vi "Grab and Attributes Setup with Save.vi"(8 "error in":errorcluster, 10 "Set Points":dbl[](array[numeric])=[1.0, 5.0, -0.1, 50.0]) -> (0 "error out":errorcluster)   [LabVIEW 2015]
doc: "The Grab and Attributes Setup example VI allows the user to view the current attributes and settings, update attribute settings, acquire images continuously, and display the images in an image control."
uses:
  <vilib>/vision/driver/IMAQdx.llb/IMAQdx Acquisition Mode.ctl
  <vilib>/vision/driver/IMAQdx.llb/IMAQdx Buffer Number Mode.ctl
  <vilib>/userDefined/High Color/IMAQdx.ctl
panel:
  in  "Cancel":bool
  in  "OK":bool
  in  "Tab Control 2":enum32{"Configure", "Help"}(tab)
  in  "Record images":bool
  in  "Image folder":path
  in  "Image Save Rate (s)":dbl=10.0 format="%#_5f"
  out "Interface elevation":dbl
  out "Camera Name":T1
  in  "Attribute Table":string(tree)
  in  "Tab Control":T2(tab)
  in  "U32 Value Control":u32(slide) min=480 max=921600 step=1 scale=829440.0..921600.0
  in  "DBL Value Control":dbl(slide) min=0.0 max=3.999 step=1.0 scale=0.0..3.999
  in  "String Value Control":string
  in  "Enum Value Control":u32(ring) items=["160x90 I420 15.00fps", "160x90 RGB24 15.00fps", "160x100 I420 15.00fps", "160x100 RGB24 15.00fps", "160x120 I420 15.00fps", "160x120 RGB24 15.00fps", "176x144 I420 15.00fps", "176x144 RGB24 15.00fps", "320x180 I420 15.00fps", "320x180 RGB24 15.00fps", "320x200 I420 15.00fps", "320x200 RGB24 15.00fps", "320x240 I420 15.00fps", "320x240 RGB24 15.00fps", "352x288 I420 15.00fps", "352x288 RGB24 15.00fps", "640x360 I420 15.00fps", "640x360 RGB24 15.00fps", "640x400 I420 15.00fps", "640x400 RGB24 15.00fps", "640x480 I420 30.00fps", "640x480 RGB24 30.00fps", "768x480 I420 15.00fps", "768x480 RGB24 15.00fps", "800x450 I420 15.00fps", "800x450 RGB24 15.00fps", "800x500 I420 15.00fps", "800x500 RGB24 15.00fps", "800x600 I420 15.00fps", "800x600 RGB24 15.00fps", "864x480 I420 15.00fps", "864x480 RGB24 15.00fps", "960x720 I420 15.00fps", "960x720 RGB24 15.00fps", "1280x720 I420 5.00fps", "1280x720 RGB24 5.00fps", "1280x800 I420 5.00fps", "1280x800 RGB24 5.00fps", "1280x1024 I420 5.00fps", "1280x1024 RGB24 5.00fps"]
  in  "Boolean Value Control":bool=TRUE
  in  "Command Value Control":bool
  out "Units":string
  out "Tooltip":string
  out "Image":T3(plugin-control)
  out "Buffer Number":u32
  out "Frame Rate":dbl(knob) scale=0.0..100.0 scale format="%.1f"
  in  "Grab":bool
  out "Tab Control Ref":T4
  # "Use the rectangle tool to define the region of interest where the floc water interface will appear.\nThe region of interest is saved in a configuration file.\n\nChoose a folder to save images during the experiment."
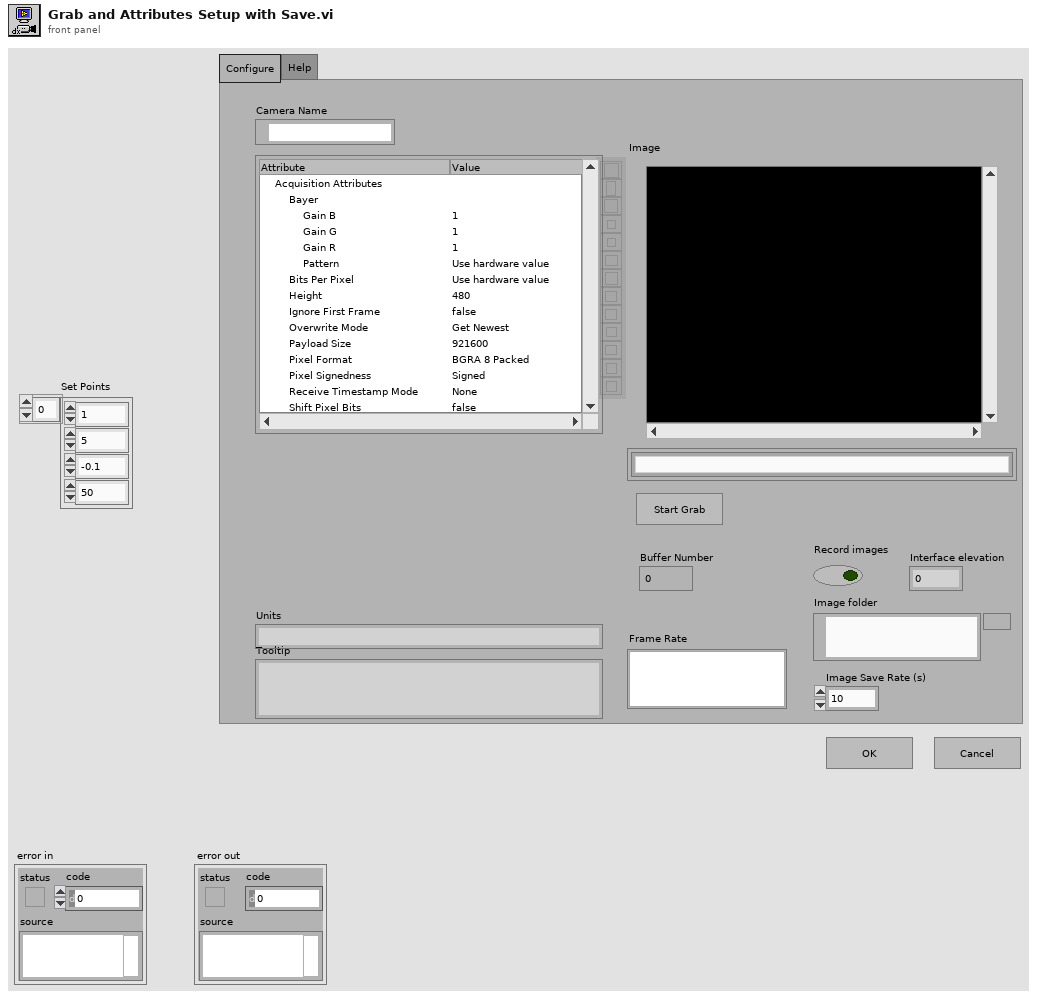
[diagram p1: front panel]
types:
  T1 = typedef "IMAQdx.ctl" = refnum<k21>
  T2 = enum32{"U32", "DBL", "String", "Enum", "Bool", "Command"}
  T3 = typedef "IMAQ Image.ctl" = refnum<image>
  T4 = cluster{"Tab Control":refnum<vi>, "U32 Value Control":refnum<vi>, "DBL Value Control":refnum<vi>, "String Value Control":refnum<vi>, "Enum Value Control":refnum<vi>, "Boolean Value Control":refnum<vi>, "Command Value Control":refnum<vi>}
  T5 = typedef "NI_Vision_Acquisition_Software.lvlib/IMAQdx Acquisition Mode.ctl" = enum32{"One Shot", "Continuous"}
  T6 = cluster{"Global Rectangle":i32[], "Contours":cluster{"Contour Type":u32, "ROI Type":u32, "Points":i32[]}[]}
  T7 = cluster{"Type":u32, "Version":u32, "Flags":u32, "SerialNumberHigh":u32, "SerialNumberLow":u32, "BusType":u32, "InterfaceName":string, "VendorName":string, "ModelName":string, "CameraFileName":string, "CameraAttributeURL":string}[]
  T8 = cluster{"Set Points[0]":dbl, "Set Points[1]":dbl, "Set Points[2]":dbl, "Set Points[3]":dbl}
  T9 = cluster{"Type":u32, "Version":u32, "Flags":u32, "SerialNumberHigh":u32, "SerialNumberLow":u32, "BusType":u32, "InterfaceName":string, "VendorName":string, "ModelName":string, "CameraFileName":string, "CameraAttributeURL":string}
  T10 = enum8{"Enabled", "Disabled", "Disabled and Grayed Out"}
  T11 = typedef "NI_Vision_Acquisition_Software.lvlib/IMAQdx Buffer Number Mode.ctl" = enum32{"Next", "Last", "Buffer Number"}
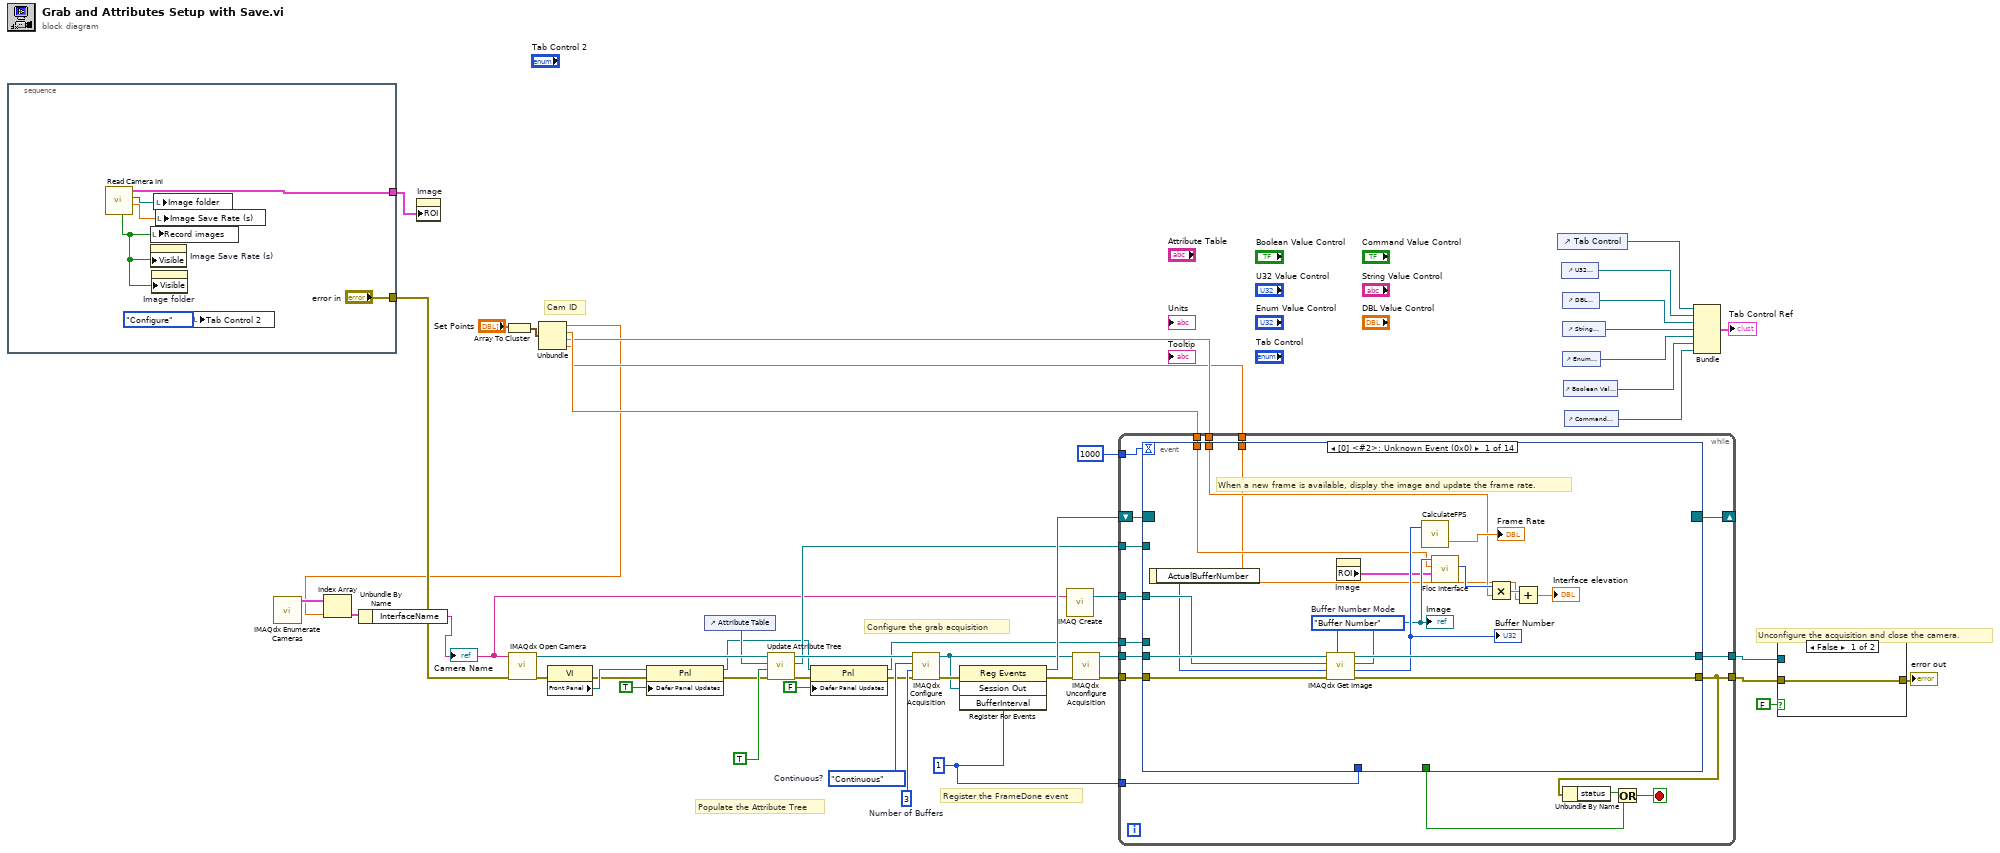
[diagram p0: block diagram]
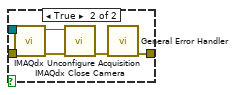
[diagram p2: hidden frame]
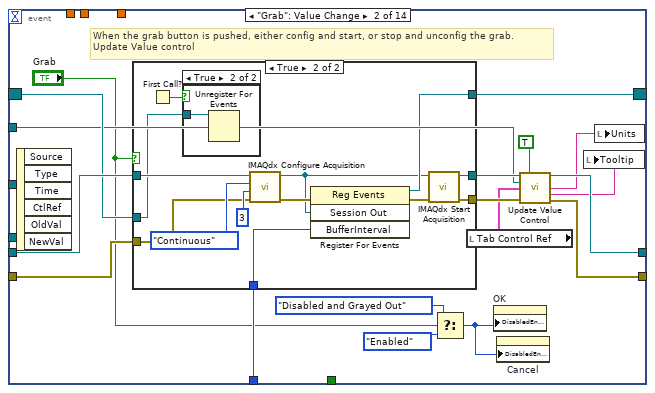
[diagram p3: hidden frame]
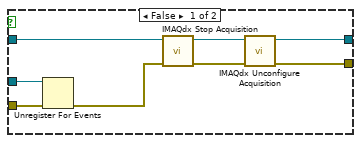
[diagram p4: hidden frame]
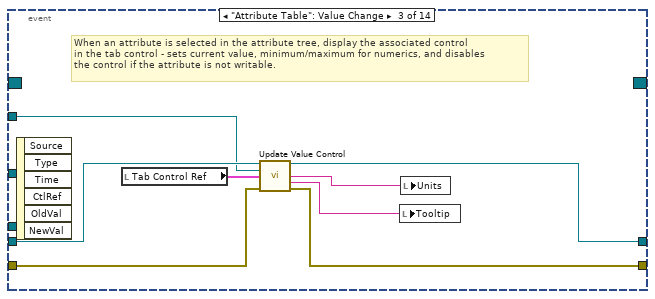
[diagram p6: hidden frame]
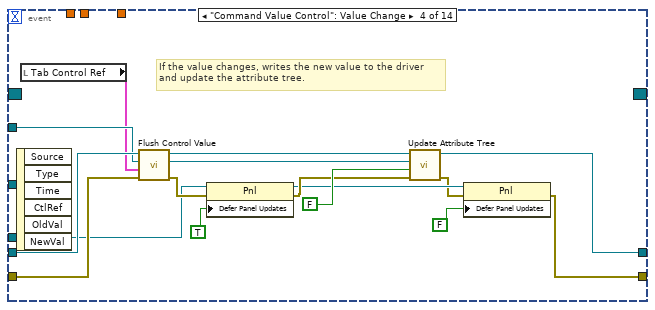
[diagram p7: hidden frame]
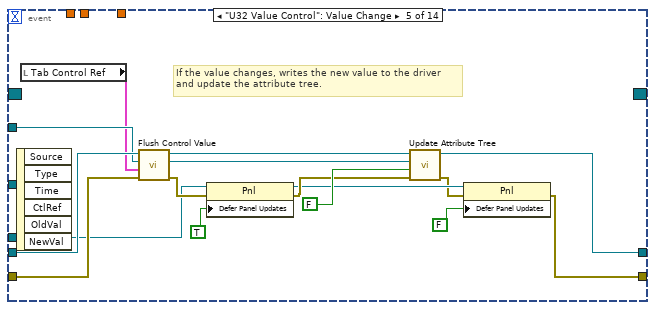
[diagram p8: hidden frame]
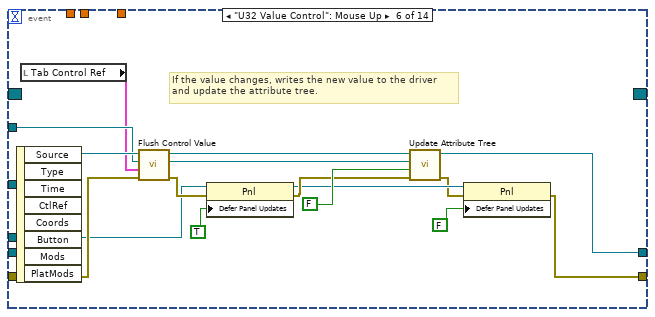
[diagram p9: hidden frame]
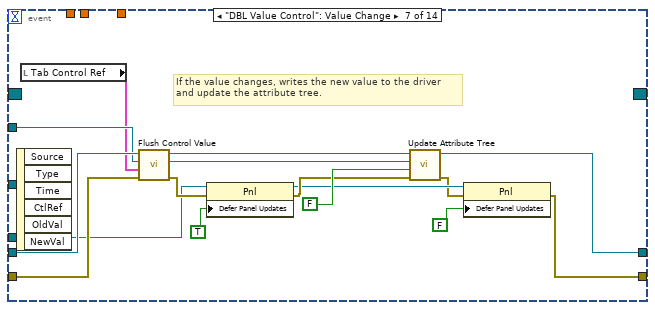
[diagram p10: hidden frame]
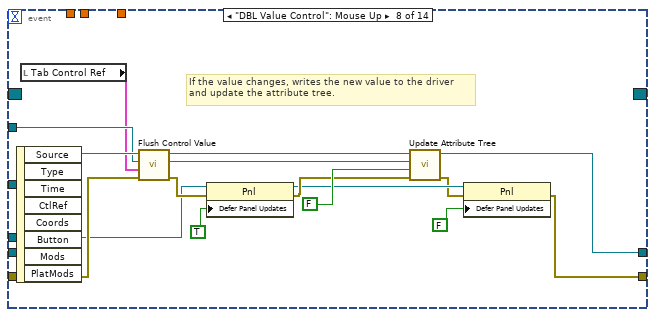
[diagram p11: hidden frame]
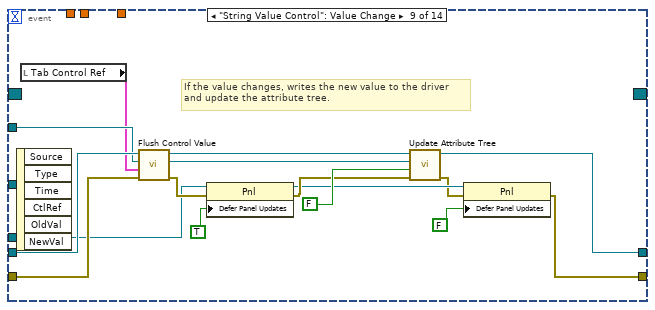
[diagram p12: hidden frame]
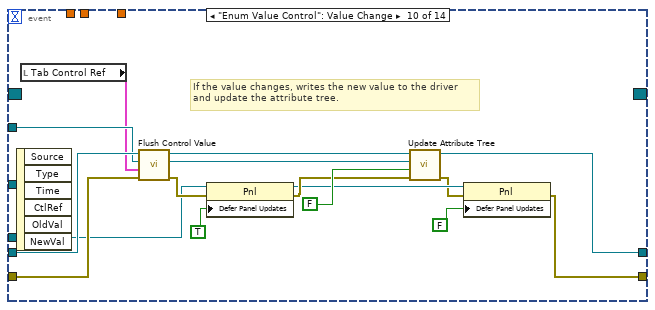
[diagram p13: hidden frame]
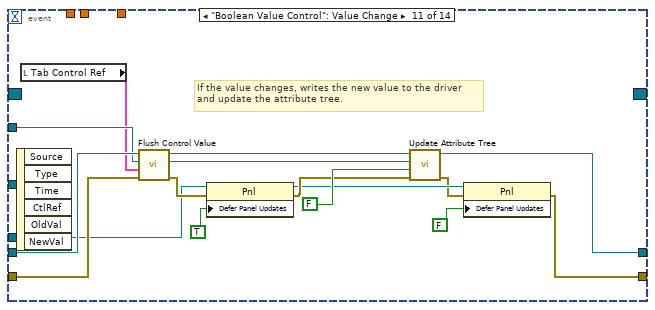
[diagram p14: hidden frame]
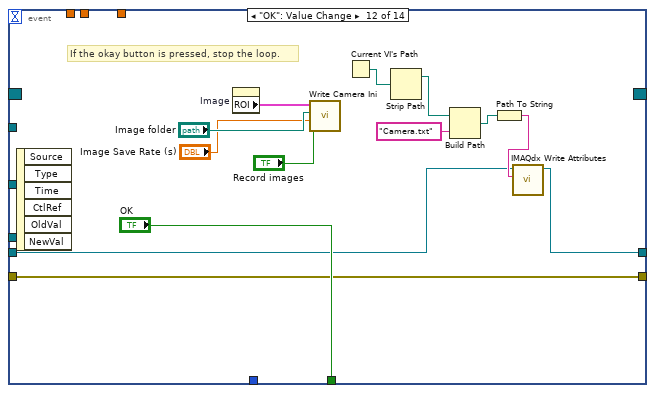
[diagram p15: hidden frame]
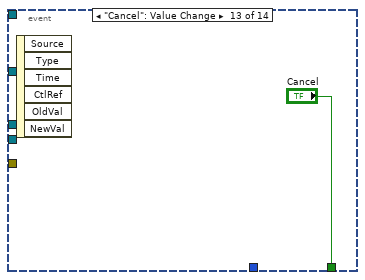
[diagram p16: hidden frame]
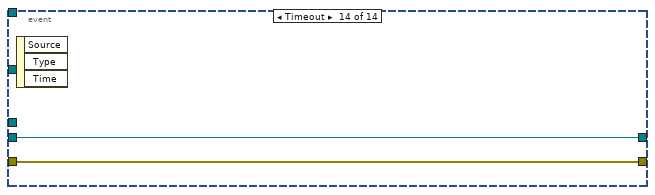
[diagram p17: hidden frame]
diagram:
  w20 = u32 1 ("BufferInterval")
  w47 = u32 3  # Number of Buffers
  w48 = IMAQdx_Acquisition_Mode."Continuous"  # Continuous?
  # "Cam ID"
  # "Unconfigure the acquisition and close the camera."
  # "Register the FrameDone event"
  # "Configure the grab acquisition"
  # "Populate the Attribute Tree"
  n1 = stacked-sequence {
    tunnel: [w55] -> w10
    tunnel: ["error in"] -> w9
    frame #0 {
      n2 = call "Read Camera Ini.vi"() -> ("Image Save Rate (s)"=w52:dbl, "Image folder"=w53:path, "ROI"=w55:T6, "Record images"=w50:bool)  [unwired: 7 in, 1 out]
      n3 = local write "Record images"(w50) -> ()
      n4 = property on="Image Save Rate (s)" class="DigNum (strict)"("Visible"=w50) -> ()  [unwired: 2 in, 2 out]
      n5 = property on="Image folder" class="Path"("Visible"=w50) -> ()  [unwired: 2 in, 2 out]
      n6 = local write "Image folder"(w53) -> ()
      n7 = local write "Image Save Rate (s)"(w52) -> ()
      n8 = local write "Tab Control 2"(enum32{"Configure", "Help"}."Configure" ("Tab Control")) -> ()
    }
  }
  n9 = call <vilib>:"IMAQdx Enumerate Cameras.vi"() -> ("Camera Information Array"=w8:T7)  [unwired: 10 in, 1 out]
  n10 = property on="Image" class="ImageControl"("ROI"=w10) -> ()  [unwired: 2 in, 2 out]
  n11 = Array To Cluster(array="Set Points") -> (cluster=w15:T8)
  n12 = Unbundle(w15) -> ("Set Points[0]"=w7:dbl, "Set Points[1]"=w13:dbl, "Set Points[2]"=w12:dbl, "Set Points[3]"=w11:dbl)
  n13 = Index Array(array=w8, index=w7) -> (element=w6:T9)
  n14 = Unbundle By Name(w6) -> ("InterfaceName"=w5:string)
  "Camera Name" <- w5
  n15 = call <vilib>:"IMAQdx Open Camera.vi"("error in"=w9, "Session In"=w5) -> ("error out"=w21:errorcluster, "Session Out"=w35:T1)  [unwired: 1 in, 7 out]
  n16 = property class="VI"(error in=w21) -> (error out=w22:errorcluster, "Front Panel"=w23:refnum<vi>)  [unwired: 1 in, 1 out]
  n17 = property class="Pnl"(reference=w23, error in=w22, "Defer Panel Updates"=TRUE) -> (reference out=w26:refnum<vi>, error out=w30:errorcluster)
  n18 = control-ref of="Attribute Table"() -> (w33:refnum<vi>)
  n19 = call "Update Attribute Tree.vi"("error in"=w30, "Flush Tree?"=TRUE, "Tree Control In"=w33, "Camera Name In"=w35) -> ("error out"=w29:errorcluster, "Tree Control Out"=w31:refnum<vi>, "Session Out"=w34:T1)  [unwired: 1 out]
  n20 = property class="Pnl"(reference=w26, error in=w29, "Defer Panel Updates"=FALSE) -> (reference out=w25:refnum<vi>, error out=w27:errorcluster)
  n21 = call <vilib>:"IMAQdx Configure Acquisition.vi"("error in"=w27, "Number of Buffers"=w47, "Continuous?"=w48, "Session In"=w34) -> ("error out"=w46:errorcluster, "Session Out"=w17:T1)  [unwired: 6 out]
  n22 = register-events(error in=w46, w17, w20) -> (reference out=w45:refnum<event-registration>, error out=w19:errorcluster)  [unwired: 1 in]
  n23 = call "IMAQ Create"("Image Name"=w5) -> ("New Image"=w49:T3)  [unwired: 3 in, 2 out]
  n24 = call <vilib>:"IMAQdx Unconfigure Acquisition.vi"("error in"=w19, "Session In"=w17) -> ("error out"=w18:errorcluster, "Session Out"=w16:T1)  [unwired: 8 out]
  n25 = while {
    tunnel: [w67] -> w4
    tunnel: w18 -> [w69]
    tunnel: w16 -> [w70]
    tunnel: [w66] -> w3
    tunnel: w49 -> [w68]
    tunnel: 1000 -> [w64]
    tunnel: w31 -> [w63]
    tunnel: w25 -> [w62]
    tunnel: w20 -> [w60]
    shift-right: [w59] -> _
    shift-left: w45 -> [w65]
    tunnel: w13 -> [w58]
    tunnel: w12 -> [w57]
    tunnel: w11 -> [w56]
    stop <- w72 stop-if-true
    n26 = event shown="[0] <#2>: Unknown Event (0x0)" {
      selector: w65 -> [_ w104 _ _ _ _ _ _ _ _ _ _ _ _]
      dyn-events: [_ w106 _ _ _ _ _ _ _ _ _ _ _ _] -> w59
      timeout: w64 -> [_ _ _ _ _ _ _ _ _ _ _ _ _ _]
      tunnel: w70 -> [w89 w107 w137 w152 w168 w184 w200 w216 w232 w248 w264 w267 _ w280]
      tunnel: w69 -> [w88 w103 w135 w153 w169 w185 w201 w217 w233 w249 w265 w277 _ w281]
      tunnel: w68 -> [w87 _ _ _ _ _ _ _ _ _ _ _ _ _]
      tunnel: [w86 w101 w136 w138 w154 w170 w186 w202 w218 w234 w250 w266 _ w280] -> w67
      tunnel: [w85 w99 w134 w139 w155 w171 w187 w203 w219 w235 w251 w277 _ w281] -> w66
      tunnel: w63 -> [_ w97 w130 w150 w166 w182 w198 w214 w230 w246 w262 _ _ _]
      tunnel: w62 -> [_ _ _ w144 w160 w176 w192 w208 w224 w240 w256 _ _ _]
      tunnel: [_ _ _ _ _ _ _ _ _ _ _ "OK" "Cancel" _] -> w61
      tunnel: w60 -> [_ w105 _ _ _ _ _ _ _ _ _ _ _ _]
      tunnel: w58 -> [w76 _ _ _ _ _ _ _ _ _ _ _ _ _]
      tunnel: w57 -> [w75 _ _ _ _ _ _ _ _ _ _ _ _ _]
      tunnel: w56 -> [w74 _ _ _ _ _ _ _ _ _ _ _ _ _]
      event event type 1.21.x0 {
        w83 = IMAQdx_Buffer_Number_Mode."Buffer Number"  # Buffer Number Mode
        # "When a new frame is available, display the image and update the frame rate."
        n27 = event-data() -> ("ActualBufferNumber"=w82:u32)  [unwired: 1 out]
        n28 = call <vilib>:"IMAQdx Get Image.vi"("Buffer Number Mode (Next)"=w83, "error in"=w88, "Buffer Number In"=w82, "Image In"=w87, "Session In"=w89) -> ("error out"=w85:errorcluster, "Buffer Number Out"=w81:u32, "Image Out"=w80:T3, "Session Out"=w86:T1)  [unwired: 3 out]
        "Image" <- w80
        "Buffer Number" <- w81
        n29 = property on="Image" class="ImageControl"() -> ("ROI"=w73:T6)  [unwired: 2 in, 2 out]
        n30 = call "CalculateFPS.vi"("buffer number"=w81) -> ("processed FPS"=→"Frame Rate":dbl)  [unwired: 2 out]
        n31 = call "Floc Interface.vi"("ROI"=w73, "Smooth Length"=w76, "Image"=w80) -> ("min index"=w77:i32)  [unwired: 4 in, 4 out]
        n32 = Multiply(x=w77, y=w75) -> (x*y=w79:dbl)
        n33 = Add(x=w79, y=w74) -> (x+y=→"Interface elevation":dbl)
      }
      event "Grab": Value Change {
        # "When the grab button is pushed, either config and start, or stop and unconfig the grab.\nUpdate Value control"
        n34 = event-data() -> ()  [unwired: 7 out]
        n35 = case shown="True" "Grab" {
          tunnel: w107 -> [w115 w126]
          tunnel: [w112 w128] -> w102
          tunnel: [w111 w127] -> w100
          tunnel: [_ w121] -> w106
          tunnel: w105 -> [_ w119]
          tunnel: w104 -> [w110 w117]
          tunnel: w103 -> [w108 w118]
          frame False {
            n36 = Unregister For Events(event registration refnum=w110, error in=w108) -> (error out=w109:errorcluster)
            n37 = call <vilib>:"IMAQdx Stop Acquisition.vi"("error in"=w109, "Session In"=w115) -> ("error out"=w113:errorcluster, "Session Out"=w114:T1)  [unwired: 8 out]
            n38 = call <vilib>:"IMAQdx Unconfigure Acquisition.vi"("error in"=w113, "Session In"=w114) -> ("error out"=w111:errorcluster, "Session Out"=w112:T1)  [unwired: 8 out]
          }
          frame True {
            n39 = First Call?() -> (First Call?: T/F=w116:bool)
            n40 = case shown="True" w116 {
              tunnel: w117 -> [_ w129]
              frame False {
              }
              frame True {
                n41 = Unregister For Events(event registration refnum=w129) -> ()  [unwired: 1 in, 1 out]
              }
            }
            n42 = call <vilib>:"IMAQdx Configure Acquisition.vi"("error in"=w118, "Number of Buffers"=u32 3, "Continuous?"=IMAQdx_Acquisition_Mode."Continuous", "Session In"=w126) -> ("error out"=w123:errorcluster, "Session Out"=w120:T1)  [unwired: 6 out]
            n43 = register-events(error in=w123, w120, w119) -> (reference out=w121:refnum<event-registration>, error out=w122:errorcluster)  [unwired: 1 in]
            n44 = call <vilib>:"IMAQdx Start Acquisition.vi"("error in"=w122, "Session In"=w120) -> ("error out"=w127:errorcluster, "Session Out"=w128:T1)  [unwired: 8 out]
          }
        }
        n45 = Select(t=T10."Disabled and Grayed Out" ("Disabled"), s="Grab", f=T10."Enabled" ("Disabled")) -> (s? t:f=w93:T10)
        n46 = local read "Tab Control Ref"() -> (w98:T4)
        n47 = property on="OK" class="Bool"("DisabledEnum"=w93) -> ()  [unwired: 2 in, 2 out]
        n48 = property on="Cancel" class="Bool"("DisabledEnum"=w93) -> ()  [unwired: 2 in, 2 out]
        n49 = call "Update Value Control.vi"("Session In"=w102, "Force update?"=TRUE, "Tree Control In"=w97, "Tab Control Ref In"=w98, "error in (no error)"=w100) -> ("Session Out"=w101:T1, "Units"=w96:string, "Tooltip"=w95:string, "error out"=w99:errorcluster)  [unwired: 7 out]
        n50 = local write "Tooltip"(w95) -> ()
        n51 = local write "Units"(w96) -> ()
      }
      event "Attribute Table": Value Change {
        # "When an attribute is selected in the attribute tree, display the associated control\nin the tab control - sets current value, minimum/maximum for numerics, and disables\nthe control if the attribute is not writable."
        n52 = event-data() -> ()  [unwired: 7 out]
        n53 = local read "Tab Control Ref"() -> (w133:T4)
        n54 = call "Update Value Control.vi"("Session In"=w137, "Tree Control In"=w130, "Tab Control Ref In"=w133, "error in (no error)"=w135) -> ("Session Out"=w136:T1, "Units"=w132:string, "Tooltip"=w131:string, "error out"=w134:errorcluster)  [unwired: 1 in, 7 out]
        n55 = local write "Tooltip"(w131) -> ()
        n56 = local write "Units"(w132) -> ()
      }
      event "Command Value Control": Value Change {
        # "If the value changes, writes the new value to the driver\nand update the attribute tree."
        n57 = event-data() -> ()  [unwired: 7 out]
        n58 = local read "Tab Control Ref"() -> (w149:T4)
        n59 = call "Flush Control Value.vi"("error in (no error)"=w153, "Tab Control Ref In"=w149, "Tree Control In"=w150, "Session In"=w152) -> ("error out"=w145:errorcluster, "Tree Control Out"=w148:refnum<vi>, "Session Out"=w151:T1)  [unwired: 1 out]
        n60 = property class="Pnl"(reference=w144, error in=w145, "Defer Panel Updates"=TRUE) -> (reference out=w142:refnum<vi>, error out=w146:errorcluster)
        n61 = call "Update Attribute Tree.vi"("error in"=w146, "Flush Tree?"=FALSE, "Tree Control In"=w148, "Camera Name In"=w151) -> ("error out"=w141:errorcluster, "Session Out"=w138:T1)  [unwired: 2 out]
        n62 = property class="Pnl"(reference=w142, error in=w141, "Defer Panel Updates"=FALSE) -> (error out=w139:errorcluster)  [unwired: 1 out]
      }
      event "U32 Value Control": Value Change {
        # "If the value changes, writes the new value to the driver\nand update the attribute tree."
        n63 = event-data() -> ()  [unwired: 7 out]
        n64 = local read "Tab Control Ref"() -> (w165:T4)
        n65 = call "Flush Control Value.vi"("error in (no error)"=w169, "Tab Control Ref In"=w165, "Tree Control In"=w166, "Session In"=w168) -> ("error out"=w161:errorcluster, "Tree Control Out"=w164:refnum<vi>, "Session Out"=w167:T1)  [unwired: 1 out]
        n66 = property class="Pnl"(reference=w160, error in=w161, "Defer Panel Updates"=TRUE) -> (reference out=w158:refnum<vi>, error out=w162:errorcluster)
        n67 = call "Update Attribute Tree.vi"("error in"=w162, "Flush Tree?"=FALSE, "Tree Control In"=w164, "Camera Name In"=w167) -> ("error out"=w157:errorcluster, "Session Out"=w154:T1)  [unwired: 2 out]
        n68 = property class="Pnl"(reference=w158, error in=w157, "Defer Panel Updates"=FALSE) -> (error out=w155:errorcluster)  [unwired: 1 out]
      }
      event "U32 Value Control": Mouse Up {
        # "If the value changes, writes the new value to the driver\nand update the attribute tree."
        n69 = event-data() -> ()  [unwired: 9 out]
        n70 = local read "Tab Control Ref"() -> (w181:T4)
        n71 = call "Flush Control Value.vi"("error in (no error)"=w185, "Tab Control Ref In"=w181, "Tree Control In"=w182, "Session In"=w184) -> ("error out"=w177:errorcluster, "Tree Control Out"=w180:refnum<vi>, "Session Out"=w183:T1)  [unwired: 1 out]
        n72 = property class="Pnl"(reference=w176, error in=w177, "Defer Panel Updates"=TRUE) -> (reference out=w174:refnum<vi>, error out=w178:errorcluster)
        n73 = call "Update Attribute Tree.vi"("error in"=w178, "Flush Tree?"=FALSE, "Tree Control In"=w180, "Camera Name In"=w183) -> ("error out"=w173:errorcluster, "Session Out"=w170:T1)  [unwired: 2 out]
        n74 = property class="Pnl"(reference=w174, error in=w173, "Defer Panel Updates"=FALSE) -> (error out=w171:errorcluster)  [unwired: 1 out]
      }
      event "DBL Value Control": Value Change {
        # "If the value changes, writes the new value to the driver\nand update the attribute tree."
        n75 = event-data() -> ()  [unwired: 7 out]
        n76 = local read "Tab Control Ref"() -> (w197:T4)
        n77 = call "Flush Control Value.vi"("error in (no error)"=w201, "Tab Control Ref In"=w197, "Tree Control In"=w198, "Session In"=w200) -> ("error out"=w193:errorcluster, "Tree Control Out"=w196:refnum<vi>, "Session Out"=w199:T1)  [unwired: 1 out]
        n78 = property class="Pnl"(reference=w192, error in=w193, "Defer Panel Updates"=TRUE) -> (reference out=w190:refnum<vi>, error out=w194:errorcluster)
        n79 = call "Update Attribute Tree.vi"("error in"=w194, "Flush Tree?"=FALSE, "Tree Control In"=w196, "Camera Name In"=w199) -> ("error out"=w189:errorcluster, "Session Out"=w186:T1)  [unwired: 2 out]
        n80 = property class="Pnl"(reference=w190, error in=w189, "Defer Panel Updates"=FALSE) -> (error out=w187:errorcluster)  [unwired: 1 out]
      }
      event "DBL Value Control": Mouse Up {
        # "If the value changes, writes the new value to the driver\nand update the attribute tree."
        n81 = event-data() -> ()  [unwired: 9 out]
        n82 = local read "Tab Control Ref"() -> (w213:T4)
        n83 = call "Flush Control Value.vi"("error in (no error)"=w217, "Tab Control Ref In"=w213, "Tree Control In"=w214, "Session In"=w216) -> ("error out"=w209:errorcluster, "Tree Control Out"=w212:refnum<vi>, "Session Out"=w215:T1)  [unwired: 1 out]
        n84 = property class="Pnl"(reference=w208, error in=w209, "Defer Panel Updates"=TRUE) -> (reference out=w206:refnum<vi>, error out=w210:errorcluster)
        n85 = call "Update Attribute Tree.vi"("error in"=w210, "Flush Tree?"=FALSE, "Tree Control In"=w212, "Camera Name In"=w215) -> ("error out"=w205:errorcluster, "Session Out"=w202:T1)  [unwired: 2 out]
        n86 = property class="Pnl"(reference=w206, error in=w205, "Defer Panel Updates"=FALSE) -> (error out=w203:errorcluster)  [unwired: 1 out]
      }
      event "String Value Control": Value Change {
        # "If the value changes, writes the new value to the driver\nand update the attribute tree."
        n87 = event-data() -> ()  [unwired: 7 out]
        n88 = local read "Tab Control Ref"() -> (w229:T4)
        n89 = call "Flush Control Value.vi"("error in (no error)"=w233, "Tab Control Ref In"=w229, "Tree Control In"=w230, "Session In"=w232) -> ("error out"=w225:errorcluster, "Tree Control Out"=w228:refnum<vi>, "Session Out"=w231:T1)  [unwired: 1 out]
        n90 = property class="Pnl"(reference=w224, error in=w225, "Defer Panel Updates"=TRUE) -> (reference out=w222:refnum<vi>, error out=w226:errorcluster)
        n91 = call "Update Attribute Tree.vi"("error in"=w226, "Flush Tree?"=FALSE, "Tree Control In"=w228, "Camera Name In"=w231) -> ("error out"=w221:errorcluster, "Session Out"=w218:T1)  [unwired: 2 out]
        n92 = property class="Pnl"(reference=w222, error in=w221, "Defer Panel Updates"=FALSE) -> (error out=w219:errorcluster)  [unwired: 1 out]
      }
      event "Enum Value Control": Value Change {
        # "If the value changes, writes the new value to the driver\nand update the attribute tree."
        n93 = event-data() -> ()  [unwired: 7 out]
        n94 = local read "Tab Control Ref"() -> (w245:T4)
        n95 = call "Flush Control Value.vi"("error in (no error)"=w249, "Tab Control Ref In"=w245, "Tree Control In"=w246, "Session In"=w248) -> ("error out"=w241:errorcluster, "Tree Control Out"=w244:refnum<vi>, "Session Out"=w247:T1)  [unwired: 1 out]
        n96 = property class="Pnl"(reference=w240, error in=w241, "Defer Panel Updates"=TRUE) -> (reference out=w238:refnum<vi>, error out=w242:errorcluster)
        n97 = call "Update Attribute Tree.vi"("error in"=w242, "Flush Tree?"=FALSE, "Tree Control In"=w244, "Camera Name In"=w247) -> ("error out"=w237:errorcluster, "Session Out"=w234:T1)  [unwired: 2 out]
        n98 = property class="Pnl"(reference=w238, error in=w237, "Defer Panel Updates"=FALSE) -> (error out=w235:errorcluster)  [unwired: 1 out]
      }
      event "Boolean Value Control": Value Change {
        # "If the value changes, writes the new value to the driver\nand update the attribute tree."
        n99 = event-data() -> ()  [unwired: 7 out]
        n100 = local read "Tab Control Ref"() -> (w261:T4)
        n101 = call "Flush Control Value.vi"("error in (no error)"=w265, "Tab Control Ref In"=w261, "Tree Control In"=w262, "Session In"=w264) -> ("error out"=w257:errorcluster, "Tree Control Out"=w260:refnum<vi>, "Session Out"=w263:T1)  [unwired: 1 out]
        n102 = property class="Pnl"(reference=w256, error in=w257, "Defer Panel Updates"=TRUE) -> (reference out=w254:refnum<vi>, error out=w258:errorcluster)
        n103 = call "Update Attribute Tree.vi"("error in"=w258, "Flush Tree?"=FALSE, "Tree Control In"=w260, "Camera Name In"=w263) -> ("error out"=w253:errorcluster, "Session Out"=w250:T1)  [unwired: 2 out]
        n104 = property class="Pnl"(reference=w254, error in=w253, "Defer Panel Updates"=FALSE) -> (error out=w251:errorcluster)  [unwired: 1 out]
      }
      event "OK": Value Change {
        # "If the okay button is pressed, stop the loop."
        n105 = event-data() -> ()  [unwired: 7 out]
        n106 = property on="Image" class="ImageControl"() -> ("ROI"=w276:T6)  [unwired: 2 in, 2 out]
        n107 = call "Write Camera Ini.vi"("Record images"="Record images", "Image Save Rate (s)"="Image Save Rate (s)", "Image folder"="Image folder", "ROI"=w276) -> ()  [unwired: 8 in]
        n108 = Current VI's Path() -> (path=w269:path)
        n109 = Strip Path(path=w269) -> (stripped path=w270:path)  [unwired: 1 out]
        n110 = Build Path(base path=w270, name or relative path="Camera.txt") -> (appended path=w272:path)
        n111 = Path To String(path=w272) -> (string=w268:string)
        n112 = call <vilib>:"IMAQdx Write Attributes.vi"("Filename"=w268, "Session In"=w267) -> ("Session Out"=w266:T1)  [unwired: 8 in, 1 out]
      }
      event "Cancel": Value Change {
        n113 = event-data() -> ()  [unwired: 7 out]
      }
      event Timeout {
        n114 = event-data() -> ()  [unwired: 4 out]
      }
    }
    n115 = Unbundle By Name(w66) -> ("status"=w71:bool)
    n116 = Or(x=w71, y=w61) -> (x .or. y?=w72:bool)
  }
  n117 = control-ref of="Tab Control"() -> (w43:refnum<vi>)
  n118 = control-ref of="U32 Value Control"() -> (w41:refnum<vi>)
  n119 = control-ref of="DBL Value Control"() -> (w40:refnum<vi>)
  n120 = control-ref of="String Value Control"() -> (w42:refnum<vi>)
  n121 = control-ref of="Enum Value Control"() -> (w39:refnum<vi>)
  n122 = control-ref of="Boolean Value Control"() -> (w38:refnum<vi>)
  n123 = control-ref of="Command Value Control"() -> (w37:refnum<vi>)
  n124 = Bundle("Tab Control"=w43, "U32 Value Control"=w41, "DBL Value Control"=w40, "String Value Control"=w42, "Enum Value Control"=w39, "Boolean Value Control"=w38, "Command Value Control"=w37) -> (→"Tab Control Ref":T4)  [unwired: 1 out]
  n125 = case shown="False" FALSE {
    tunnel: w4 -> [_ w286]
    tunnel: w3 -> [w282 w285]
    tunnel: [w282 w283] -> w2
    frame False {
    }
    frame True {
      n126 = call <vilib>:"IMAQdx Unconfigure Acquisition.vi"("error in"=w285, "Session In"=w286) -> ("error out"=w288:errorcluster, "Session Out"=w287:T1)  [unwired: 8 out]
      n127 = call <vilib>:"IMAQdx Close Camera.vi"("error in"=w288, "Session In"=w287) -> ("error out"=w284:errorcluster)  [unwired: 9 out]
      n128 = call <vilib>:"General Error Handler.vi"("error in (no error)"=w284) -> ("error out"=w283:errorcluster)  [unwired: 2 in, 12 out]
    }
  }
  "error out" <- w2
